vi "xwpfDocument Tests Read.vi"() -> ()   [LabVIEW 2017, in "Word_Specific.lvlib"]
uses:
  src/LabVIEW NPOI/Word_Specific.lvlib
  src/LabVIEW NPOI/xwpfDocument/xwpfDocument.lvclass/xwpfDocument.ctl
  src/LabVIEW NPOI/xwpfDocument/Get Elements.Text.vi
  src/LabVIEW NPOI/xwpfDocument/Get Headers.Text.vi
  src/LabVIEW NPOI/xwpfDocument/Get Paragraphs.Text.vi
  src/LabVIEW NPOI/xwpfDocument/Get Footers.Text.vi
  src/LabVIEW NPOI/xwpfDocument/Get Tables.Text.vi
  src/LabVIEW NPOI/xwpfDocument.Element/xwpfDocument.Element.lvclass
  src/LabVIEW NPOI/xwpfDocument/xwpfDocument.lvclass
panel:
  out "Elements":string[](array[string])
  out "Tables.Text":string[][][](array[string])
  out "Footers:Text":string[](array[string])
  out "Paragraphs.Text":string[](array[string])
  out "Headers.Text":string[](array[string])
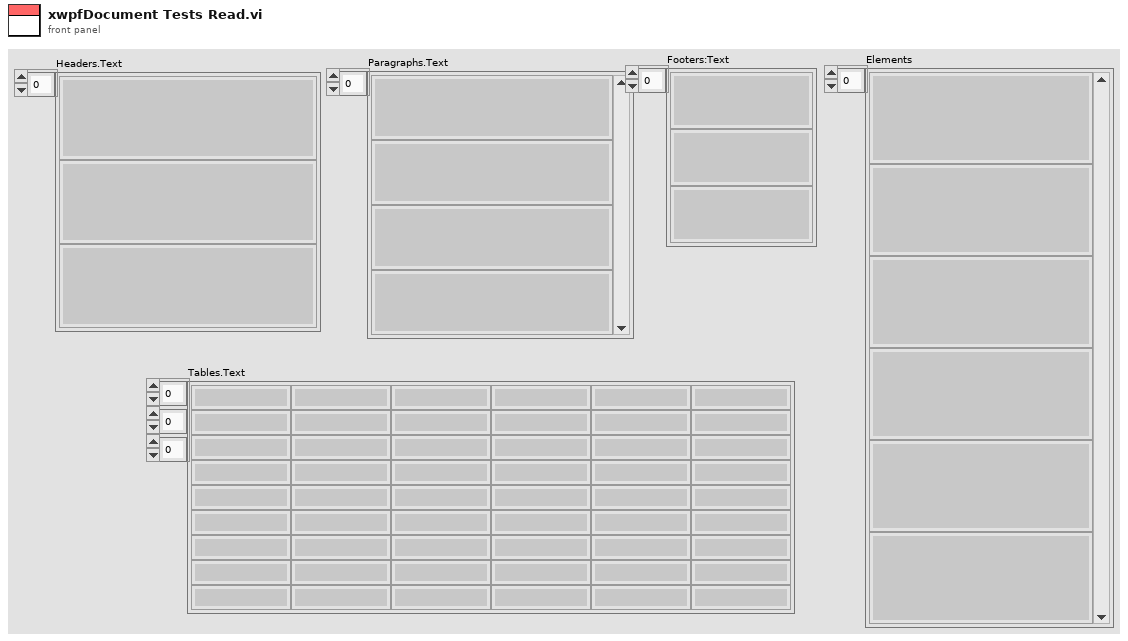
[diagram p1: front panel]
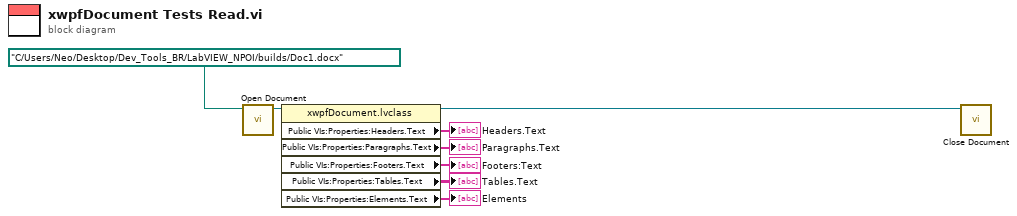
[diagram p0: block diagram]
diagram:
  n1 = call "Open Document.vi"("Document Path"=path "C:/Users/Neo/Desktop/Dev_Tools_BR/LabVIEW_NPOI/builds/Doc1.docx") -> ("xwpfDocument out"=w8:refnum<class "xwpfDocument.lvclass">)  [unwired: 9 in, 1 out]
  n2 = property class="xwpfDocument.lvclass"(reference=w8) -> (reference out=w3:refnum<class "xwpfDocument.lvclass">, "Public VIs:Properties:Headers.Text"=→"Headers.Text":string[], "Public VIs:Properties:Paragraphs.Text"=→"Paragraphs.Text":string[], "Public VIs:Properties:Footers.Text"=→"Footers:Text":string[], "Public VIs:Properties:Tables.Text"=→"Tables.Text":string[][][], "Public VIs:Properties:Elements.Text"=→"Elements":string[])  [unwired: 1 in, 1 out]
  n3 = call "Close Document.vi"("xwpfDocument in"=w3) -> ()  [unwired: 9 in, 2 out]
